vi "vna get measurement catalog.vi"(8 "error in (no error)":errorcluster, 11 "VISA resource name":refnum<visa-resource-name>) -> (0 "error out":errorcluster, 2 "measurements":cluster{"name":string, "param":string}[](array[cluster]), 3 "VISA resource name 2":refnum<visa-resource-name>)   [LabVIEW 2013]
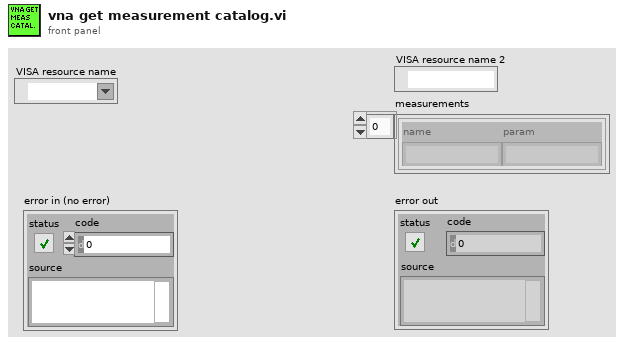
[diagram p1: front panel]
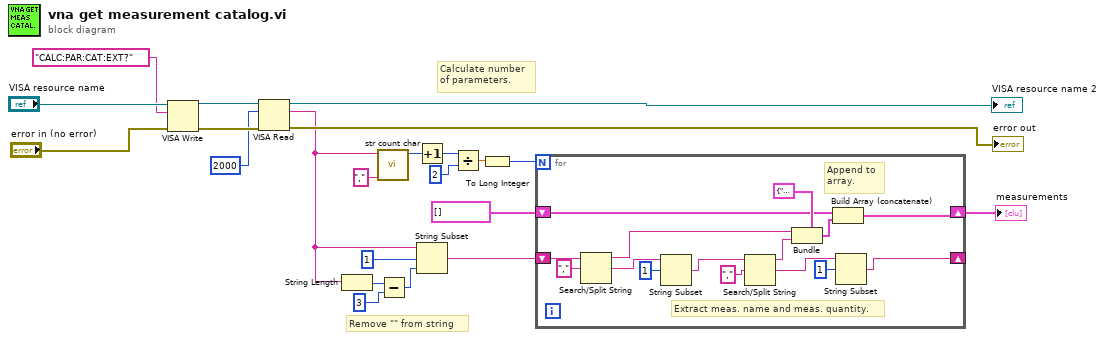
[diagram p0: block diagram]
diagram:
  # "Calculate number\nof parameters."
  # "Remove \"\" from string"
  n1 = VISA Write(VISA resource name="VISA resource name", write buffer="CALC:PAR:CAT:EXT?", error in (no error)="error in (no error)") -> (VISA resource name out=w19:refnum<visa-resource-name>, error out=w18:errorcluster)  [unwired: 1 out]
  n2 = VISA Read(VISA resource name=w19, byte count=u32 2000, error in (no error)=w18) -> (VISA resource name out=→"VISA resource name 2":refnum<visa-resource-name>, read buffer=w5:string, error out=→"error out":errorcluster)  [unwired: 1 out]
  n3 = String Length(string=w5) -> (length=w4:i32)
  n4 = call "str count char.vi"("search char"=",", "input string"=w5) -> ("occurences"=w15:i64)  [unwired: 9 in]
  n5 = Subtract(x=w4, y=3) -> (x-y=w2:i32)
  n6 = Increment(x=w15) -> (x+1=w14:i64)
  n7 = String Subset(string=w5, offset (0)=1 ("length (rest)"), length (rest)=w2) -> (substring=w1:string)
  n8 = Divide(x=w14, y=i64 2) -> (x/y=w10:dbl)
  n9 = To Long Integer(number=w10) -> (32bit integer=w9:i32)
  n10 = for {
    N: w9 -> [_]
    shift-right: [w31] -> w7
    shift-left: cluster{"name":string, "param":string}[] [] ("measurements") -> [w30]
    shift-right: [w23] -> _
    shift-left: w1 -> [w37]
    # "Append to\narray."
    # "Extract meas. name and meas. quantity."
    n11 = Search/Split String(string=w37, search string/char (-)=",") -> (substring before match=w35:string, match + rest of string=w28:string)  [unwired: 1 in, 1 out]
    n12 = String Subset(string=w28, offset (0)=1) -> (substring=w26:string)  [unwired: 1 in]
    n13 = Search/Split String(string=w26, search string/char (-)=",") -> (substring before match=w33:string, match + rest of string=w25:string)  [unwired: 1 in, 1 out]
    n14 = Bundle(cluster=cluster{"name":string, "param":string} {"name"="", "param"=""} ("Cluster"), "name"=w35, "param"=w33) -> (w29:cluster{"name":string, "param":string})
    n15 = Build Array (concatenate)(w30, w29) -> (w31:cluster{"name":string, "param":string}[])
    n16 = String Subset(string=w25, offset (0)=1) -> (substring=w23:string)  [unwired: 1 in]
  }
  "measurements" <- w7
